vi "Control AlgorithmPID.vi"(5 "Motor to Control":dbl, 8 "Manual Control":bool, 9 "Angles In":dbl[](array[numeric]), 10 "JoystickIn":i16[](array[numeric])) -> (2 "Target Angles":dbl[](array[numeric]), 3 "MotorsOut":u16[](array[numeric]))   [LabVIEW 2012, in "ProcessorHelperFunctions.lvlib"]
uses:
  ProcessorHelperFunctions.lvlib
panel:
  in  "D gain":dbl
  in  "I Gain":dbl
  in  "Pgain":dbl=1.5
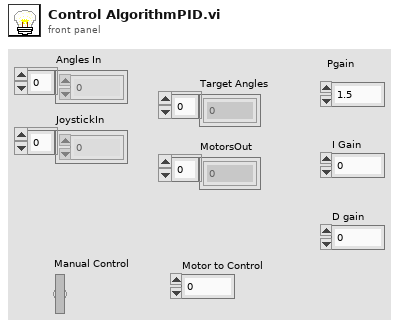
[diagram p1: front panel]
types:
  T1 = cluster{"JoystickIn[0]":i16, "JoystickIn[1]":i16, "JoystickIn[2]":i16, "JoystickIn[3]":i16, "JoystickIn[4]":i16, "JoystickIn[5]":i16, "JoystickIn[6]":i16, "JoystickIn[7]":i16, "JoystickIn[8]":i16, "JoystickIn[9]":i16}
  T2 = cluster{"Angles In[0]":dbl, "Angles In[1]":dbl, "Angles In[2]":dbl, "Angles In[3]":dbl}
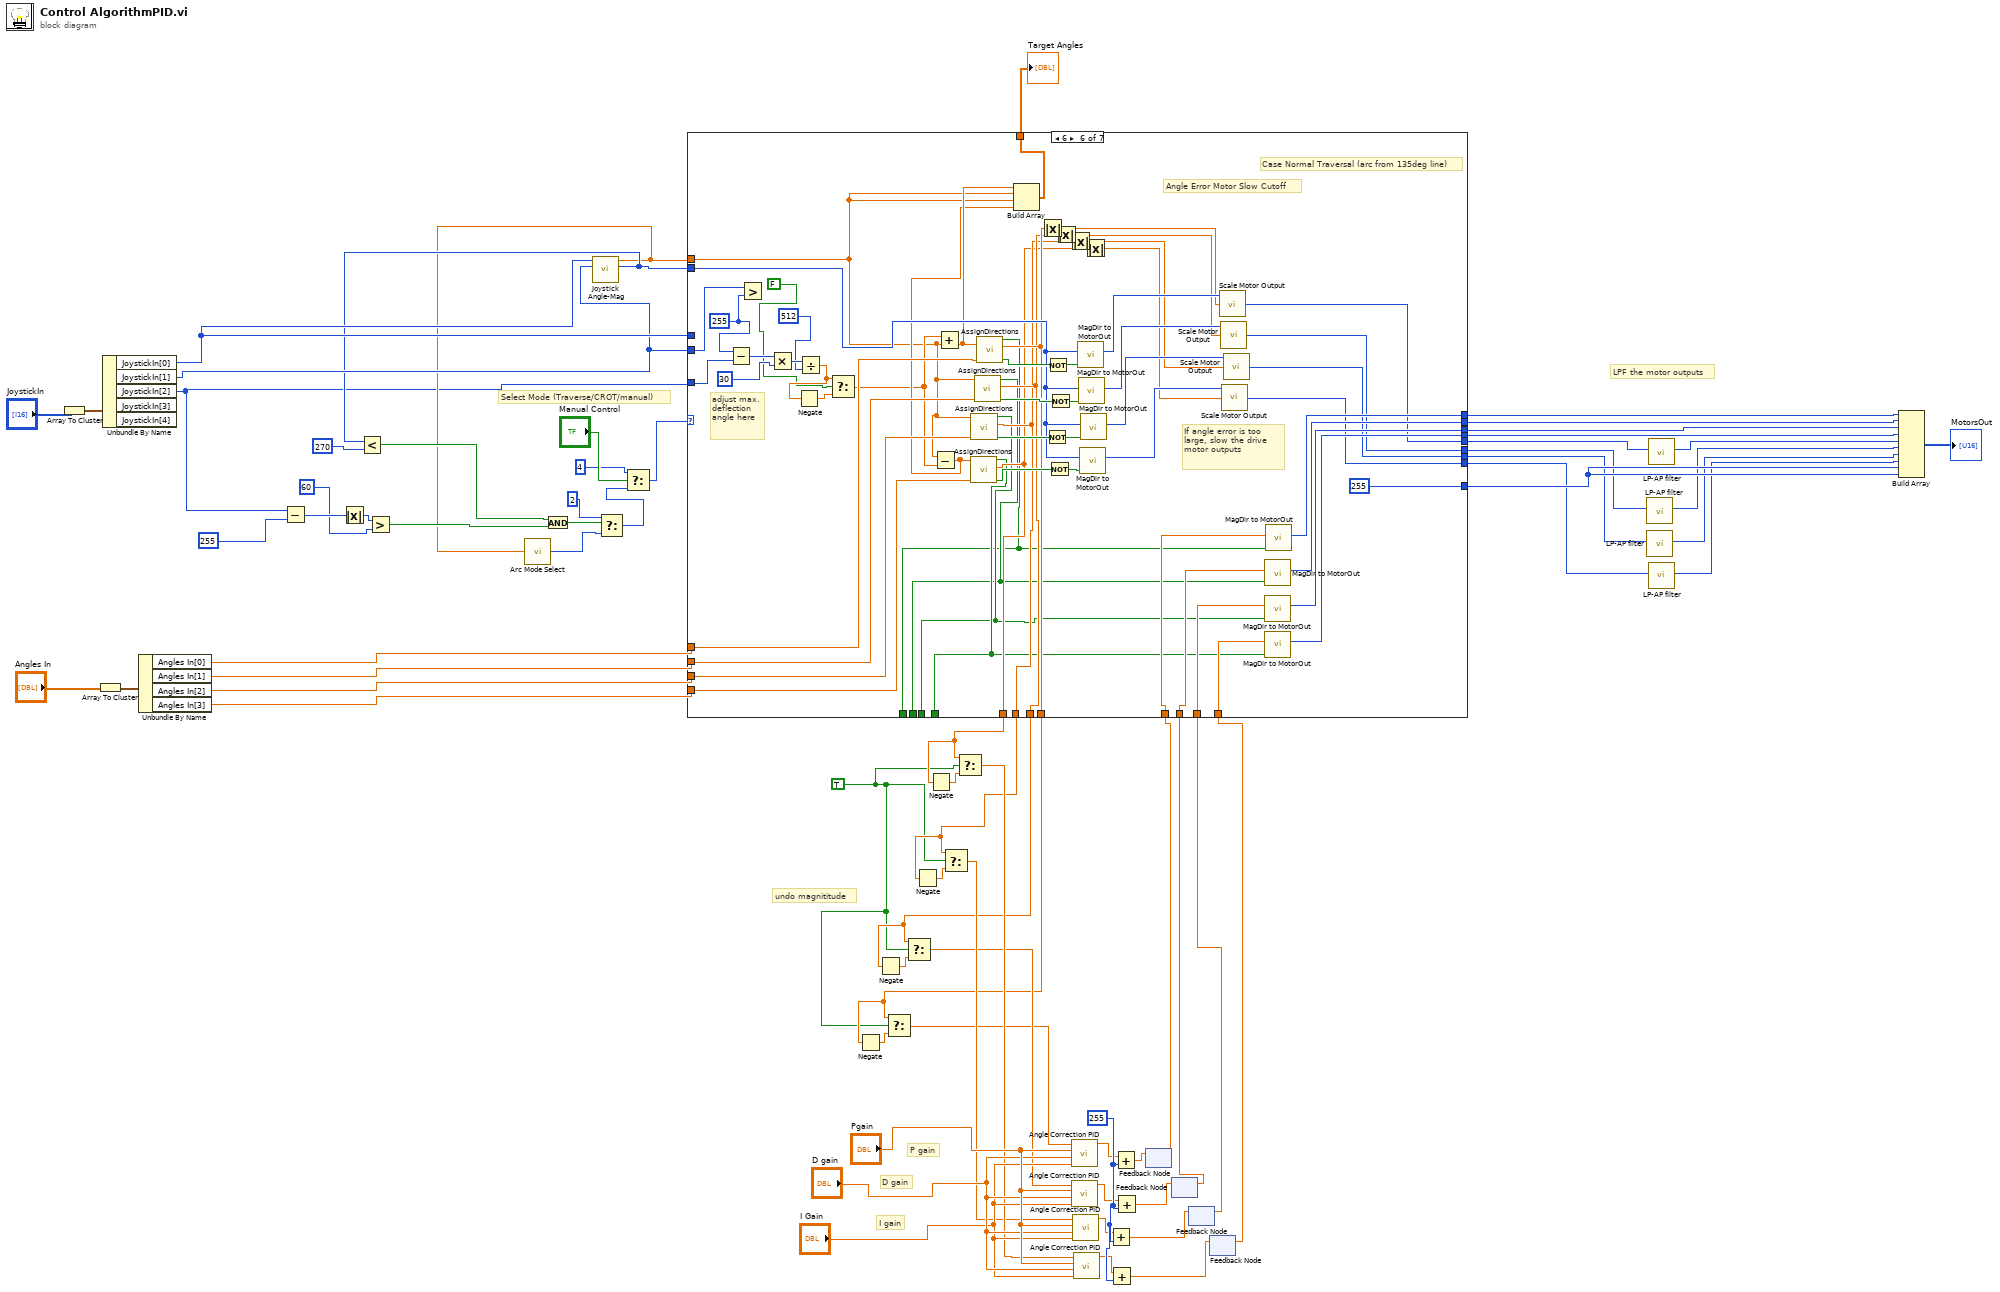
[diagram p0: block diagram]
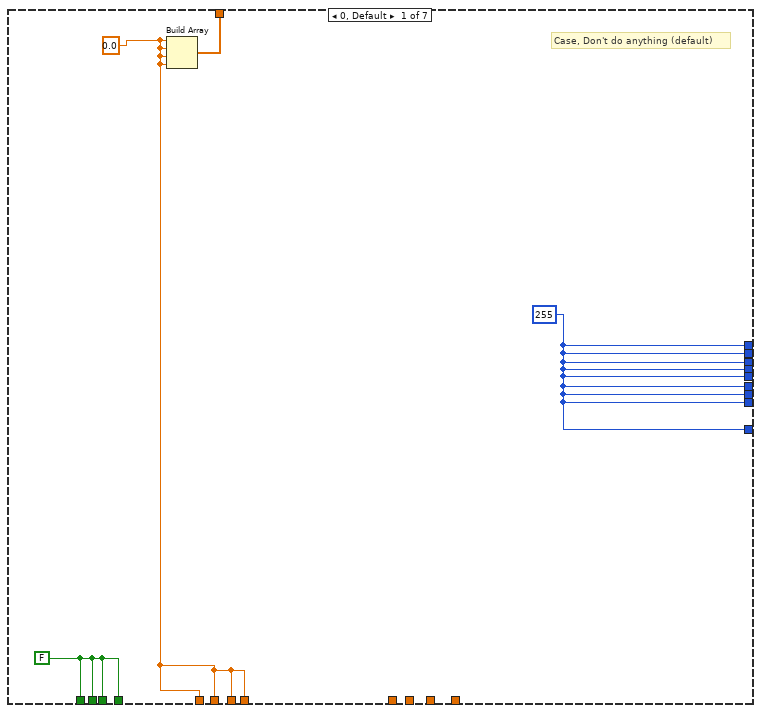
[diagram p2: hidden frame]
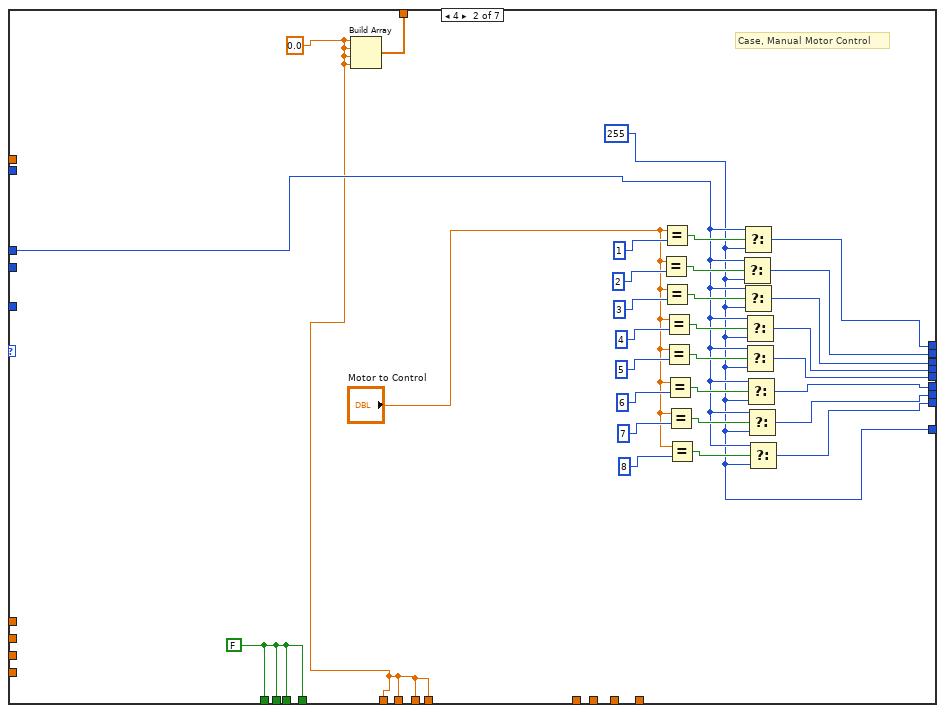
[diagram p3: hidden frame]
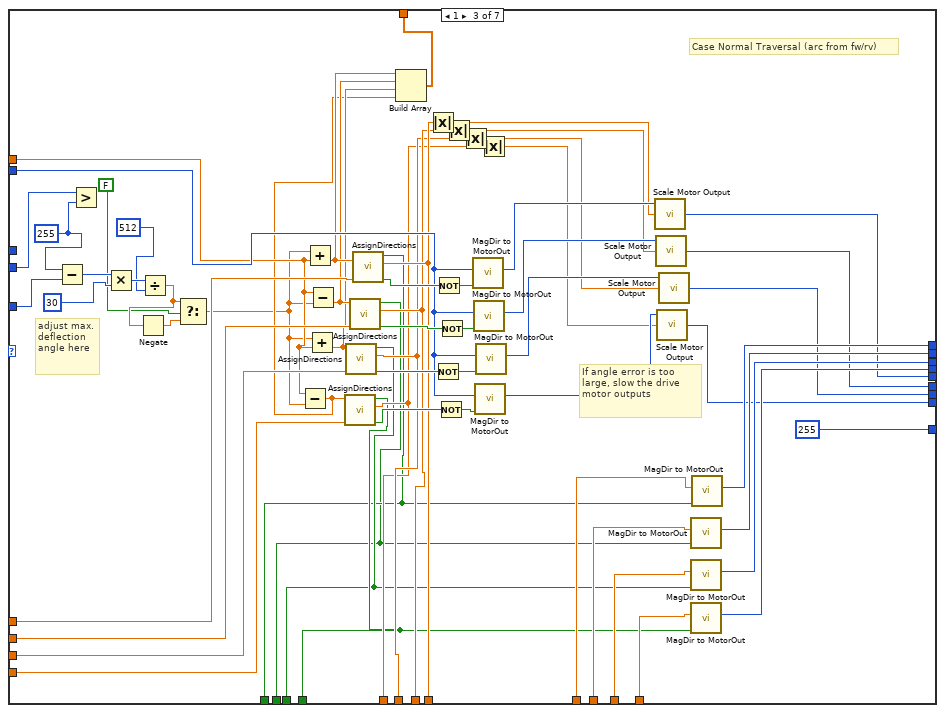
[diagram p4: hidden frame]
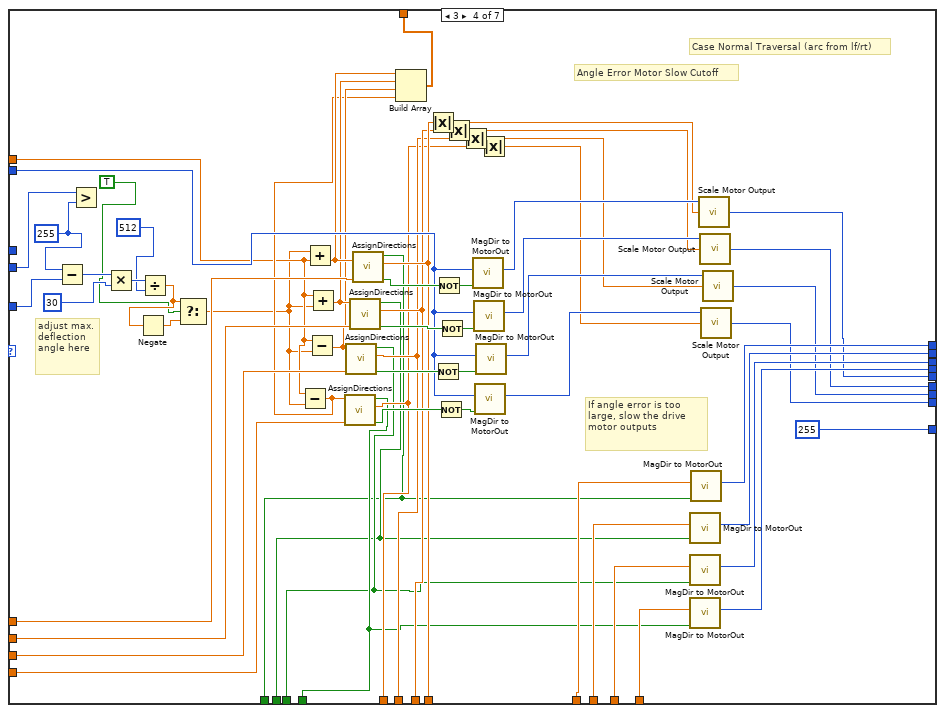
[diagram p5: hidden frame]
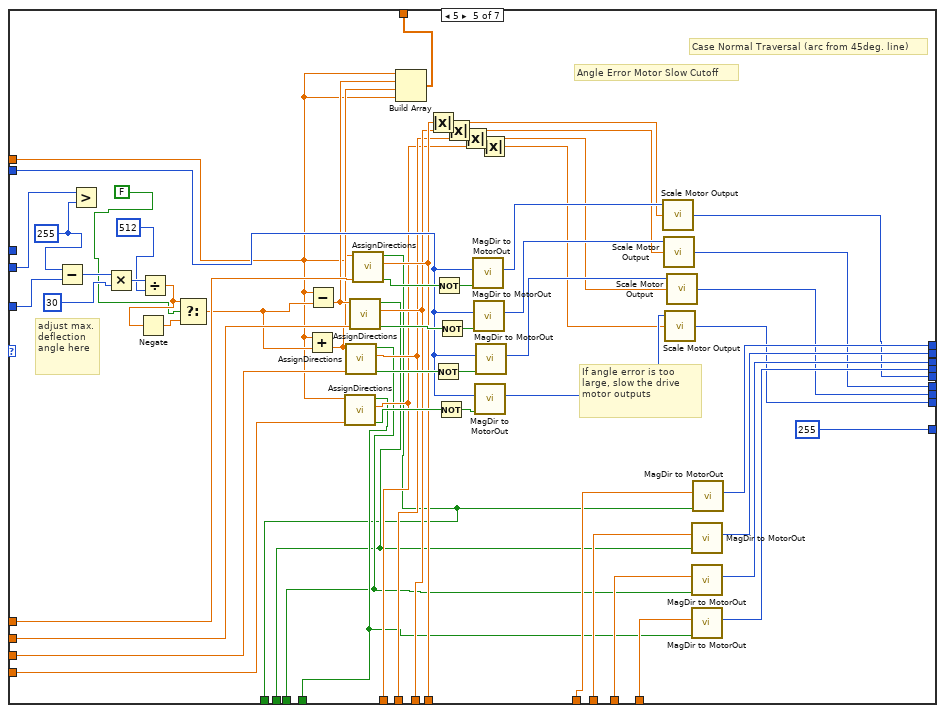
[diagram p6: hidden frame]
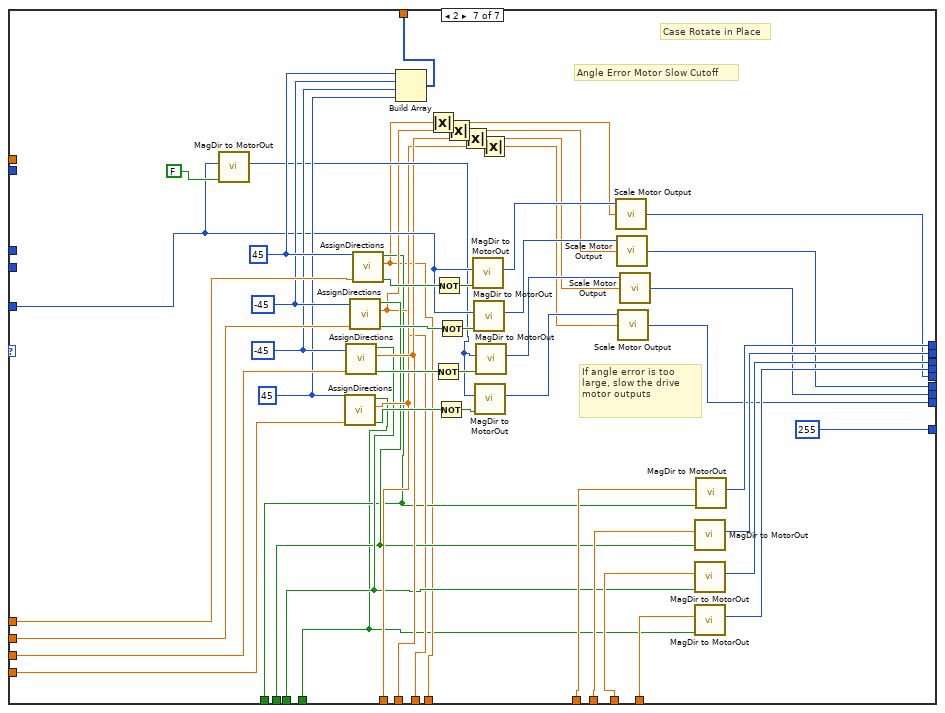
[diagram p7: hidden frame]
diagram:
  w6 = TRUE
  w30 = 255
  # "undo magnititude"
  # "I gain"
  # "D gain"
  # "P gain"
  # "LPF the motor outputs"
  # "Select Mode (Traverse/CROT/manual)"
  n1 = Array To Cluster(array="JoystickIn") -> (cluster=w70:T1)
  n2 = Array To Cluster(array="Angles In") -> (cluster=w63:T2)
  n3 = Unbundle By Name(w70) -> ("JoystickIn[0]"=w57:i16, "JoystickIn[1]"=w47:i16, "JoystickIn[2]"=w1:i16)  [unwired: 2 out]
  n4 = Unbundle By Name(w63) -> ("Angles In[0]"=w61:dbl, "Angles In[1]"=w60:dbl, "Angles In[2]"=w59:dbl, "Angles In[3]"=w58:dbl)
  n5 = Subtract(x=w1, y=255) -> (x-y=w54:i32)
  n6 = Absolute Value(x=w54) -> (abs(x)=w53:i32)
  n7 = Greater?(x=w53, y=60) -> (0:w49:bool)
  n8 = call "Joystick Angle-Mag.vi"("Yaxis"=w47, "Xaxis"=w57) -> ("Mag"=w33:i16, "Angle"=w31:dbl)  [unwired: 8 in]
  n9 = Less?(x=w33, y=270) -> (x < y?=w48:bool)
  n10 = call "Arc Mode Select.vi"("Angle"=w31) -> ("Mode"=w32:u8)
  n11 = And(x=w48, y=w49) -> (x .and. y?=w50:bool)
  n12 = Select(t=2, s=w50, f=w32) -> (s? t:f=w44:i32)
  n13 = Select(t=4, s="Manual Control", f=w44) -> (s? t:f=w45:i32)
  n14 = feedback #1() -> (w5:dbl)  [unwired: 1 in]
  n15 = feedback #2() -> (w4:dbl)  [unwired: 1 in]
  n16 = feedback #3() -> (w3:dbl)  [unwired: 1 in]
  n17 = feedback #4() -> (w2:dbl)  [unwired: 1 in]
  n18 = case shown="6" w45 {
    tunnel: [w75 w102 w160 w219 w276 w333 w382] -> w68
    tunnel: [w75 w86 w159 w218 w275 w332 w381] -> w67
    tunnel: [w75 w85 w158 w217 w274 w331 w380] -> w66
    tunnel: [w75 w84 w157 w216 w273 w330 w379] -> w65
    tunnel: [w75 w79 255 255 255 255 255] -> w64
    tunnel: [w75 w83 w110 w169 w227 w285 w343] -> w41
    tunnel: [w75 w82 w109 w168 w224 w284 w342] -> w39
    tunnel: [w75 w81 w108 w167 w226 w283 w345] -> w37
    tunnel: [w75 w80 w107 w166 w225 w282 w344] -> w35
    tunnel: w61 -> [_ _ w147 w206 w263 w320 w369]
    tunnel: w60 -> [_ _ w146 w205 w262 w319 w368]
    tunnel: w59 -> [_ _ w145 w204 w261 w318 w367]
    tunnel: w58 -> [_ _ w144 w203 w260 w317 w366]
    tunnel: w31 -> [_ _ w136 w187 w245 w303 _]
    tunnel: w33 -> [_ _ w143 w202 w259 w316 _]
    tunnel: w57 -> [_ w87 _ _ _ _ _]
    tunnel: w47 -> [_ _ w127 w188 w247 w302 _]
    tunnel: w1 -> [_ _ w141 w200 w257 w314 w360]
    tunnel: [w74 w105 w142 w201 w258 w315 w358] -> w56
    tunnel: [w73 w77 w125 w184 w243 w300 w339] -> w7
    tunnel: [w73 w77 w124 w183 w242 w299 w349] -> w11
    tunnel: [w73 w77 w123 w182 w241 w298 w357] -> w14
    tunnel: [w73 w77 w122 w181 w240 w297 w356] -> w17
    tunnel: w5 -> [_ _ w121 w180 w239 w296 w355]
    tunnel: w4 -> [_ _ w120 w179 w238 w295 w354]
    tunnel: w3 -> [_ _ w119 w178 w237 w294 w353]
    tunnel: w2 -> [_ _ w118 w177 w236 w293 w352]
    tunnel: [w72 w76 w117 w176 w235 w292 w338] -> _
    tunnel: [w72 w76 w116 w175 w234 w291 w351] -> _
    tunnel: [w72 w76 w114 w174 w233 w290 w350] -> _
    tunnel: [w72 w76 w115 w173 w232 w289 w348] -> _
    frame 0, Default {
      w72 = FALSE
      w73 = 0.0
      w75 = 255
      # "Case, Don't do anything (default)"
      n19 = Build Array(w73, w73, w73, w73) -> (w74:dbl[])
    }
    frame 4 {
      w76 = FALSE
      w79 = 255
      w77 = 0.0
      # "Case, Manual Motor Control"
      n20 = Build Array(w77, w77, w77, w77) -> (w105:dbl[])
      n21 = Equal?(x="Motor to Control", y=2) -> (x = y?=w100:bool)
      n22 = Equal?(x="Motor to Control", y=1) -> (x = y?=w103:bool)
      n23 = Equal?(x="Motor to Control", y=3) -> (x = y?=w98:bool)
      n24 = Equal?(x="Motor to Control", y=4) -> (x = y?=w96:bool)
      n25 = Equal?(x="Motor to Control", y=5) -> (x = y?=w94:bool)
      n26 = Equal?(x="Motor to Control", y=6) -> (x = y?=w92:bool)
      n27 = Equal?(x="Motor to Control", y=7) -> (x = y?=w90:bool)
      n28 = Equal?(x="Motor to Control", y=8) -> (x = y?=w88:bool)
      n29 = Select(t=w87, s=w100, f=w79) -> (s? t:f=w86:i32)
      n30 = Select(t=w87, s=w103, f=w79) -> (s? t:f=w102:i32)
      n31 = Select(t=w87, s=w98, f=w79) -> (s? t:f=w85:i32)
      n32 = Select(t=w87, s=w96, f=w79) -> (s? t:f=w84:i32)
      n33 = Select(t=w87, s=w94, f=w79) -> (s? t:f=w83:i32)
      n34 = Select(t=w87, s=w92, f=w79) -> (s? t:f=w82:i32)
      n35 = Select(t=w87, s=w90, f=w79) -> (s? t:f=w81:i32)
      n36 = Select(t=w87, s=w88, f=w79) -> (s? t:f=w80:i32)
    }
    frame 1 {
      w128 = 255
      # "adjust max. deflection angle here"
      # "Case Normal Traversal (arc from fw/rv)"
      # "If angle error is too large, slow the drive motor outputs"
      n37 = Subtract(x=w128, y=w141) -> (x-y=w139:i32)
      n38 = Greater?(x=w127, y=w128) -> ()  [unwired: 1 out]
      n39 = Multiply(x=w139, y=30) -> (x*y=w140:i32)
      n40 = Divide(x=w140, y=512) -> (x/y=w129:dbl)
      n41 = Negate(x=w129) -> (-x=w130:dbl)
      n42 = Select(t=w129, s=FALSE, f=w130) -> (s? t:f=w131:dbl)
      n43 = Subtract(x=w136, y=w131) -> (x-y=w132:dbl)
      n44 = Add(x=w131, y=w136) -> (x+y=w135:dbl)
      n45 = Add(x=w131, y=w136) -> (x+y=w133:dbl)
      n46 = Subtract(x=w136, y=w131) -> (x-y=w134:dbl)
      n47 = call "AssignDirections.vi"("Actual Angle"=w144, "Target Angle"=w132) -> ("Reverse Wheel Direction"=w161:bool, "Lowest Angle Error"=w122:dbl, "Turn Clockwise"=w117:bool)  [unwired: 7 in]
      n48 = call "AssignDirections.vi"("Actual Angle"=w145, "Target Angle"=w133) -> ("Reverse Wheel Direction"=w162:bool, "Lowest Angle Error"=w123:dbl, "Turn Clockwise"=w116:bool)  [unwired: 7 in]
      n49 = call "AssignDirections.vi"("Actual Angle"=w146, "Target Angle"=w134) -> ("Reverse Wheel Direction"=w163:bool, "Lowest Angle Error"=w124:dbl, "Turn Clockwise"=w114:bool)  [unwired: 7 in]
      n50 = call "AssignDirections.vi"("Actual Angle"=w147, "Target Angle"=w135) -> ("Reverse Wheel Direction"=w164:bool, "Lowest Angle Error"=w125:dbl, "Turn Clockwise"=w115:bool)  [unwired: 7 in]
      n51 = Build Array(w135, w134, w133, w132) -> (w142:dbl[])
      n52 = Absolute Value(x=w125) -> (abs(x)=w113:dbl)
      n53 = Not(x=w162) -> (.not. x?=w150:bool)
      n54 = Not(x=w164) -> (.not. x?=w148:bool)
      n55 = Not(x=w161) -> (.not. x?=w151:bool)
      n56 = Not(x=w163) -> (.not. x?=w149:bool)
      n57 = Absolute Value(x=w124) -> (abs(x)=w106:dbl)
      n58 = Absolute Value(x=w123) -> (abs(x)=w112:dbl)
      n59 = call "MagDir to MotorOut.vi"("Fwd. Dir?"=w148, "Input"=w143) -> ("Output"=w155:i16)  [unwired: 9 in]
      n60 = call "MagDir to MotorOut.vi"("Fwd. Dir?"=w149, "Input"=w143) -> ("Output"=w154:i16)  [unwired: 9 in]
      n61 = call "MagDir to MotorOut.vi"("Fwd. Dir?"=w151, "Input"=w143) -> ("Output"=w152:i16)  [unwired: 9 in]
      n62 = call "MagDir to MotorOut.vi"("Fwd. Dir?"=w150, "Input"=w143) -> ("Output"=w153:i16)  [unwired: 9 in]
      n63 = Absolute Value(x=w122) -> (abs(x)=w111:dbl)
      n64 = call "Scale Motor Output.vi"("Error Input"=w113, "Motor Input"=w155) -> ("Output"=w110:u32)  [unwired: 1 in]
      n65 = call "Scale Motor Output.vi"("Error Input"=w106, "Motor Input"=w154) -> ("Output"=w109:u32)  [unwired: 1 in]
      n66 = call "Scale Motor Output.vi"("Error Input"=w111, "Motor Input"=w152) -> ("Output"=w107:u32)  [unwired: 1 in]
      n67 = call "Scale Motor Output.vi"("Error Input"=w112, "Motor Input"=w153) -> ("Output"=w108:u32)  [unwired: 1 in]
      n68 = call "MagDir to MotorOut.vi"("Fwd. Dir?"=w114, "Input"=w120) -> ("Output"=w159:i16)  [unwired: 9 in]
      n69 = call "MagDir to MotorOut.vi"("Fwd. Dir?"=w116, "Input"=w119) -> ("Output"=w158:i16)  [unwired: 9 in]
      n70 = call "MagDir to MotorOut.vi"("Fwd. Dir?"=w117, "Input"=w118) -> ("Output"=w157:i16)  [unwired: 9 in]
      n71 = call "MagDir to MotorOut.vi"("Fwd. Dir?"=w115, "Input"=w121) -> ("Output"=w160:i16)  [unwired: 9 in]
    }
    frame 3 {
      w189 = 255
      # "adjust max. deflection angle here"
      # "Case Normal Traversal (arc from lf/rt)"
      # "Angle Error Motor Slow Cutoff"
      # "If angle error is too large, slow the drive motor outputs"
      n72 = Subtract(x=w189, y=w200) -> (x-y=w198:i32)
      n73 = Greater?(x=w188, y=w189) -> ()  [unwired: 1 out]
      n74 = Multiply(x=w198, y=30) -> (x*y=w199:i32)
      n75 = Divide(x=w199, y=512) -> (x/y=w190:dbl)
      n76 = Negate(x=w190) -> (-x=w191:dbl)
      n77 = Select(t=w190, s=TRUE, f=w191) -> (s? t:f=w186:dbl)
      n78 = Subtract(x=w187, y=w186) -> (x-y=w192:dbl)
      n79 = Add(x=w186, y=w187) -> (x+y=w195:dbl)
      n80 = Subtract(x=w187, y=w186) -> (x-y=w193:dbl)
      n81 = Add(x=w187, y=w186) -> (x+y=w194:dbl)
      n82 = call "AssignDirections.vi"("Actual Angle"=w203, "Target Angle"=w192) -> ("Reverse Wheel Direction"=w220:bool, "Lowest Angle Error"=w181:dbl, "Turn Clockwise"=w176:bool)  [unwired: 7 in]
      n83 = call "AssignDirections.vi"("Actual Angle"=w204, "Target Angle"=w193) -> ("Reverse Wheel Direction"=w221:bool, "Lowest Angle Error"=w182:dbl, "Turn Clockwise"=w175:bool)  [unwired: 7 in]
      n84 = call "AssignDirections.vi"("Actual Angle"=w205, "Target Angle"=w194) -> ("Reverse Wheel Direction"=w222:bool, "Lowest Angle Error"=w183:dbl, "Turn Clockwise"=w174:bool)  [unwired: 7 in]
      n85 = call "AssignDirections.vi"("Actual Angle"=w206, "Target Angle"=w195) -> ("Reverse Wheel Direction"=w223:bool, "Lowest Angle Error"=w184:dbl, "Turn Clockwise"=w173:bool)  [unwired: 7 in]
      n86 = Build Array(w195, w194, w193, w192) -> (w201:dbl[])
      n87 = Absolute Value(x=w184) -> (abs(x)=w172:dbl)
      n88 = Not(x=w221) -> (.not. x?=w209:bool)
      n89 = Not(x=w223) -> (.not. x?=w207:bool)
      n90 = Not(x=w220) -> (.not. x?=w210:bool)
      n91 = Not(x=w222) -> (.not. x?=w208:bool)
      n92 = Absolute Value(x=w183) -> (abs(x)=w171:dbl)
      n93 = Absolute Value(x=w182) -> (abs(x)=w170:dbl)
      n94 = call "MagDir to MotorOut.vi"("Fwd. Dir?"=w207, "Input"=w202) -> ("Output"=w214:i16)  [unwired: 9 in]
      n95 = call "MagDir to MotorOut.vi"("Fwd. Dir?"=w208, "Input"=w202) -> ("Output"=w213:i16)  [unwired: 9 in]
      n96 = call "MagDir to MotorOut.vi"("Fwd. Dir?"=w210, "Input"=w202) -> ("Output"=w211:i16)  [unwired: 9 in]
      n97 = call "MagDir to MotorOut.vi"("Fwd. Dir?"=w209, "Input"=w202) -> ("Output"=w212:i16)  [unwired: 9 in]
      n98 = Absolute Value(x=w181) -> (abs(x)=w165:dbl)
      n99 = call "MagDir to MotorOut.vi"("Fwd. Dir?"=w174, "Input"=w179) -> ("Output"=w218:i16)  [unwired: 9 in]
      n100 = call "MagDir to MotorOut.vi"("Fwd. Dir?"=w175, "Input"=w178) -> ("Output"=w217:i16)  [unwired: 9 in]
      n101 = call "MagDir to MotorOut.vi"("Fwd. Dir?"=w176, "Input"=w177) -> ("Output"=w216:i16)  [unwired: 9 in]
      n102 = call "MagDir to MotorOut.vi"("Fwd. Dir?"=w173, "Input"=w180) -> ("Output"=w219:i16)  [unwired: 9 in]
      n103 = call "Scale Motor Output.vi"("Error Input"=w172, "Motor Input"=w214) -> ("Output"=w169:u32)  [unwired: 1 in]
      n104 = call "Scale Motor Output.vi"("Error Input"=w171, "Motor Input"=w213) -> ("Output"=w168:u32)  [unwired: 1 in]
      n105 = call "Scale Motor Output.vi"("Error Input"=w165, "Motor Input"=w211) -> ("Output"=w166:u32)  [unwired: 1 in]
      n106 = call "Scale Motor Output.vi"("Error Input"=w170, "Motor Input"=w212) -> ("Output"=w167:u32)  [unwired: 1 in]
    }
    frame 5 {
      w248 = 255
      # "adjust max. deflection angle here"
      # "Case Normal Traversal (arc from 45deg. line)"
      # "Angle Error Motor Slow Cutoff"
      # "If angle error is too large, slow the drive motor outputs"
      n107 = Subtract(x=w248, y=w257) -> (x-y=w255:i32)
      n108 = Greater?(x=w247, y=w248) -> ()  [unwired: 1 out]
      n109 = Multiply(x=w255, y=30) -> (x*y=w256:i32)
      n110 = Divide(x=w256, y=512) -> (x/y=w249:dbl)
      n111 = Negate(x=w249) -> (-x=w250:dbl)
      n112 = Select(t=w249, s=FALSE, f=w250) -> (s? t:f=w246:dbl)
      n113 = Add(x=w245, y=w246) -> (x+y=w251:dbl)
      n114 = Subtract(x=w245, y=w246) -> (x-y=w252:dbl)
      n115 = call "AssignDirections.vi"("Actual Angle"=w260, "Target Angle"=w245) -> ("Reverse Wheel Direction"=w277:bool, "Lowest Angle Error"=w240:dbl, "Turn Clockwise"=w235:bool)  [unwired: 7 in]
      n116 = call "AssignDirections.vi"("Actual Angle"=w261, "Target Angle"=w251) -> ("Reverse Wheel Direction"=w278:bool, "Lowest Angle Error"=w241:dbl, "Turn Clockwise"=w234:bool)  [unwired: 7 in]
      n117 = call "AssignDirections.vi"("Actual Angle"=w262, "Target Angle"=w252) -> ("Reverse Wheel Direction"=w279:bool, "Lowest Angle Error"=w242:dbl, "Turn Clockwise"=w233:bool)  [unwired: 7 in]
      n118 = call "AssignDirections.vi"("Actual Angle"=w263, "Target Angle"=w245) -> ("Reverse Wheel Direction"=w280:bool, "Lowest Angle Error"=w243:dbl, "Turn Clockwise"=w232:bool)  [unwired: 7 in]
      n119 = Build Array(w245, w252, w251, w245) -> (w258:dbl[])
      n120 = Absolute Value(x=w243) -> (abs(x)=w231:dbl)
      n121 = Not(x=w278) -> (.not. x?=w266:bool)
      n122 = Not(x=w280) -> (.not. x?=w264:bool)
      n123 = Not(x=w277) -> (.not. x?=w267:bool)
      n124 = Not(x=w279) -> (.not. x?=w265:bool)
      n125 = Absolute Value(x=w242) -> (abs(x)=w230:dbl)
      n126 = Absolute Value(x=w241) -> (abs(x)=w229:dbl)
      n127 = call "MagDir to MotorOut.vi"("Fwd. Dir?"=w264, "Input"=w259) -> ("Output"=w271:i16)  [unwired: 9 in]
      n128 = call "MagDir to MotorOut.vi"("Fwd. Dir?"=w265, "Input"=w259) -> ("Output"=w270:i16)  [unwired: 9 in]
      n129 = call "MagDir to MotorOut.vi"("Fwd. Dir?"=w267, "Input"=w259) -> ("Output"=w268:i16)  [unwired: 9 in]
      n130 = call "MagDir to MotorOut.vi"("Fwd. Dir?"=w266, "Input"=w259) -> ("Output"=w269:i16)  [unwired: 9 in]
      n131 = Absolute Value(x=w240) -> (abs(x)=w228:dbl)
      n132 = call "Scale Motor Output.vi"("Error Input"=w231, "Motor Input"=w271) -> ("Output"=w227:u32)  [unwired: 1 in]
      n133 = call "Scale Motor Output.vi"("Error Input"=w230, "Motor Input"=w270) -> ("Output"=w224:u32)  [unwired: 1 in]
      n134 = call "Scale Motor Output.vi"("Error Input"=w228, "Motor Input"=w268) -> ("Output"=w225:u32)  [unwired: 1 in]
      n135 = call "Scale Motor Output.vi"("Error Input"=w229, "Motor Input"=w269) -> ("Output"=w226:u32)  [unwired: 1 in]
      n136 = call "MagDir to MotorOut.vi"("Fwd. Dir?"=w233, "Input"=w238) -> ("Output"=w275:i16)  [unwired: 9 in]
      n137 = call "MagDir to MotorOut.vi"("Fwd. Dir?"=w234, "Input"=w237) -> ("Output"=w274:i16)  [unwired: 9 in]
      n138 = call "MagDir to MotorOut.vi"("Fwd. Dir?"=w235, "Input"=w236) -> ("Output"=w273:i16)  [unwired: 9 in]
      n139 = call "MagDir to MotorOut.vi"("Fwd. Dir?"=w232, "Input"=w239) -> ("Output"=w276:i16)  [unwired: 9 in]
    }
    frame 6 {
      w304 = 255
      # "adjust max. deflection angle here"
      # "Case Normal Traversal (arc from 135deg line)"
      # "Angle Error Motor Slow Cutoff"
      # "If angle error is too large, slow the drive motor outputs"
      n140 = Subtract(x=w304, y=w314) -> (x-y=w312:i32)
      n141 = Greater?(x=w302, y=w304) -> ()  [unwired: 1 out]
      n142 = Multiply(x=w312, y=30) -> (x*y=w313:i32)
      n143 = Divide(x=w313, y=512) -> (x/y=w305:dbl)
      n144 = Negate(x=w305) -> (-x=w306:dbl)
      n145 = Select(t=w305, s=FALSE, f=w306) -> (s? t:f=w307:dbl)
      n146 = Subtract(x=w303, y=w307) -> (x-y=w308:dbl)
      n147 = Add(x=w307, y=w303) -> (x+y=w309:dbl)
      n148 = call "AssignDirections.vi"("Actual Angle"=w317, "Target Angle"=w308) -> ("Reverse Wheel Direction"=w334:bool, "Lowest Angle Error"=w297:dbl, "Turn Clockwise"=w292:bool)  [unwired: 7 in]
      n149 = call "AssignDirections.vi"("Actual Angle"=w318, "Target Angle"=w303) -> ("Reverse Wheel Direction"=w335:bool, "Lowest Angle Error"=w298:dbl, "Turn Clockwise"=w291:bool)  [unwired: 7 in]
      n150 = call "AssignDirections.vi"("Actual Angle"=w319, "Target Angle"=w303) -> ("Reverse Wheel Direction"=w336:bool, "Lowest Angle Error"=w299:dbl, "Turn Clockwise"=w290:bool)  [unwired: 7 in]
      n151 = call "AssignDirections.vi"("Actual Angle"=w320, "Target Angle"=w309) -> ("Reverse Wheel Direction"=w337:bool, "Lowest Angle Error"=w300:dbl, "Turn Clockwise"=w289:bool)  [unwired: 7 in]
      n152 = Build Array(w309, w303, w303, w308) -> (w315:dbl[])
      n153 = Absolute Value(x=w300) -> (abs(x)=w288:dbl)
      n154 = Not(x=w335) -> (.not. x?=w323:bool)
      n155 = Not(x=w337) -> (.not. x?=w321:bool)
      n156 = Not(x=w334) -> (.not. x?=w324:bool)
      n157 = Not(x=w336) -> (.not. x?=w322:bool)
      n158 = Absolute Value(x=w299) -> (abs(x)=w281:dbl)
      n159 = Absolute Value(x=w298) -> (abs(x)=w287:dbl)
      n160 = call "MagDir to MotorOut.vi"("Fwd. Dir?"=w321, "Input"=w316) -> ("Output"=w328:i16)  [unwired: 9 in]
      n161 = call "MagDir to MotorOut.vi"("Fwd. Dir?"=w322, "Input"=w316) -> ("Output"=w327:i16)  [unwired: 9 in]
      n162 = call "MagDir to MotorOut.vi"("Fwd. Dir?"=w324, "Input"=w316) -> ("Output"=w325:i16)  [unwired: 9 in]
      n163 = call "MagDir to MotorOut.vi"("Fwd. Dir?"=w323, "Input"=w316) -> ("Output"=w326:i16)  [unwired: 9 in]
      n164 = Absolute Value(x=w297) -> (abs(x)=w286:dbl)
      n165 = call "Scale Motor Output.vi"("Error Input"=w288, "Motor Input"=w328) -> ("Output"=w285:u32)  [unwired: 1 in]
      n166 = call "Scale Motor Output.vi"("Error Input"=w281, "Motor Input"=w327) -> ("Output"=w284:u32)  [unwired: 1 in]
      n167 = call "Scale Motor Output.vi"("Error Input"=w286, "Motor Input"=w325) -> ("Output"=w282:u32)  [unwired: 1 in]
      n168 = call "Scale Motor Output.vi"("Error Input"=w287, "Motor Input"=w326) -> ("Output"=w283:u32)  [unwired: 1 in]
      n169 = call "MagDir to MotorOut.vi"("Fwd. Dir?"=w290, "Input"=w295) -> ("Output"=w332:i16)  [unwired: 9 in]
      n170 = call "MagDir to MotorOut.vi"("Fwd. Dir?"=w291, "Input"=w294) -> ("Output"=w331:i16)  [unwired: 9 in]
      n171 = call "MagDir to MotorOut.vi"("Fwd. Dir?"=w292, "Input"=w293) -> ("Output"=w330:i16)  [unwired: 9 in]
      n172 = call "MagDir to MotorOut.vi"("Fwd. Dir?"=w289, "Input"=w296) -> ("Output"=w333:i16)  [unwired: 9 in]
    }
    frame 2 {
      w362 = 45
      w363 = -45
      w364 = -45
      w365 = 45
      # "Case Rotate in Place"
      # "Angle Error Motor Slow Cutoff"
      # "If angle error is too large, slow the drive motor outputs"
      n173 = call "MagDir to MotorOut.vi"("Fwd. Dir?"=FALSE, "Input"=w360) -> ("Output"=w359:i16)  [unwired: 9 in]
      n174 = call "AssignDirections.vi"("Actual Angle"=w366, "Target Angle"=w362) -> ("Reverse Wheel Direction"=w383:bool, "Lowest Angle Error"=w356:dbl, "Turn Clockwise"=w338:bool)  [unwired: 7 in]
      n175 = call "AssignDirections.vi"("Actual Angle"=w367, "Target Angle"=w363) -> ("Reverse Wheel Direction"=w384:bool, "Lowest Angle Error"=w357:dbl, "Turn Clockwise"=w351:bool)  [unwired: 7 in]
      n176 = call "AssignDirections.vi"("Actual Angle"=w368, "Target Angle"=w364) -> ("Reverse Wheel Direction"=w385:bool, "Lowest Angle Error"=w349:dbl, "Turn Clockwise"=w350:bool)  [unwired: 7 in]
      n177 = call "AssignDirections.vi"("Actual Angle"=w369, "Target Angle"=w365) -> ("Reverse Wheel Direction"=w386:bool, "Lowest Angle Error"=w339:dbl, "Turn Clockwise"=w348:bool)  [unwired: 7 in]
      n178 = Build Array(w365, w364, w363, w362) -> (w358:i32[])
      n179 = Absolute Value(x=w339) -> (abs(x)=w347:dbl)
      n180 = Not(x=w384) -> (.not. x?=w372:bool)
      n181 = Not(x=w386) -> (.not. x?=w370:bool)
      n182 = Not(x=w383) -> (.not. x?=w373:bool)
      n183 = Not(x=w385) -> (.not. x?=w371:bool)
      n184 = Absolute Value(x=w349) -> (abs(x)=w346:dbl)
      n185 = Absolute Value(x=w357) -> (abs(x)=w341:dbl)
      n186 = call "MagDir to MotorOut.vi"("Fwd. Dir?"=w370, "Input"=w360) -> ("Output"=w377:i16)  [unwired: 9 in]
      n187 = call "MagDir to MotorOut.vi"("Fwd. Dir?"=w371, "Input"=w360) -> ("Output"=w376:i16)  [unwired: 9 in]
      n188 = call "MagDir to MotorOut.vi"("Fwd. Dir?"=w373, "Input"=w359) -> ("Output"=w374:i16)  [unwired: 9 in]
      n189 = call "MagDir to MotorOut.vi"("Fwd. Dir?"=w372, "Input"=w359) -> ("Output"=w375:i16)  [unwired: 9 in]
      n190 = Absolute Value(x=w356) -> (abs(x)=w340:dbl)
      n191 = call "Scale Motor Output.vi"("Error Input"=w347, "Motor Input"=w377) -> ("Output"=w343:u32)  [unwired: 1 in]
      n192 = call "Scale Motor Output.vi"("Error Input"=w346, "Motor Input"=w376) -> ("Output"=w342:u32)  [unwired: 1 in]
      n193 = call "Scale Motor Output.vi"("Error Input"=w340, "Motor Input"=w374) -> ("Output"=w344:u32)  [unwired: 1 in]
      n194 = call "Scale Motor Output.vi"("Error Input"=w341, "Motor Input"=w375) -> ("Output"=w345:u32)  [unwired: 1 in]
      n195 = call "MagDir to MotorOut.vi"("Fwd. Dir?"=w350, "Input"=w354) -> ("Output"=w381:i16)  [unwired: 9 in]
      n196 = call "MagDir to MotorOut.vi"("Fwd. Dir?"=w351, "Input"=w353) -> ("Output"=w380:i16)  [unwired: 9 in]
      n197 = call "MagDir to MotorOut.vi"("Fwd. Dir?"=w338, "Input"=w352) -> ("Output"=w379:i16)  [unwired: 9 in]
      n198 = call "MagDir to MotorOut.vi"("Fwd. Dir?"=w348, "Input"=w355) -> ("Output"=w382:i16)  [unwired: 9 in]
    }
  }
  "Target Angles" <- w56
  n199 = Negate(x=w7) -> (-x=w9:dbl)
  n200 = Negate(x=w11) -> (-x=w12:dbl)
  n201 = Select(t=w7, s=w6, f=w9) -> (s? t:f=w8:dbl)
  n202 = Select(t=w11, s=w6, f=w12) -> (s? t:f=w10:dbl)
  n203 = Negate(x=w14) -> (-x=w15:dbl)
  n204 = Negate(x=w17) -> (-x=w18:dbl)
  n205 = Select(t=w14, s=w6, f=w15) -> (s? t:f=w13:dbl)
  n206 = Select(t=w17, s=w6, f=w18) -> (s? t:f=w16:dbl)
  n207 = call "Angle Correction PID.vi"("I gain"="I Gain", "D gain"="D gain", "P gain"="Pgain", "Error In"=w8) -> ("Output"=w25:dbl)  [unwired: 7 in]
  n208 = call "Angle Correction PID.vi"("I gain"="I Gain", "D gain"="D gain", "P gain"="Pgain", "Error In"=w10) -> ("Output"=w24:dbl)  [unwired: 7 in]
  n209 = call "Angle Correction PID.vi"("I gain"="I Gain", "D gain"="D gain", "P gain"="Pgain", "Error In"=w13) -> ("Output"=w23:dbl)  [unwired: 7 in]
  n210 = call "Angle Correction PID.vi"("I gain"="I Gain", "D gain"="D gain", "P gain"="Pgain", "Error In"=w16) -> ("Output"=w22:dbl)  [unwired: 7 in]
  n211 = Add(x=w23, y=w30) -> (x+y=w27:dbl)
  n212 = Add(x=w22, y=w30) -> (x+y=w26:dbl)
  n213 = Add(x=w25, y=w30) -> (x+y=w29:dbl)
  n214 = Add(x=w24, y=w30) -> (x+y=w28:dbl)
  n215 = feedback-in #1(w29) -> ()
  n216 = feedback-in #2(w28) -> ()
  n217 = feedback-in #3(w27) -> ()
  n218 = feedback-in #4(w26) -> ()
  n219 = call "LP-AP filter.vi"("Input"=w39) -> ("Output"=w38:u16)  [unwired: 9 in, 1 out]
  n220 = call "LP-AP filter.vi"("Input"=w37) -> ("Output"=w36:u16)  [unwired: 9 in, 1 out]
  n221 = call "LP-AP filter.vi"("Input"=w41) -> ("Output"=w40:u16)  [unwired: 9 in, 1 out]
  n222 = call "LP-AP filter.vi"("Input"=w35) -> ("Output"=w34:u16)  [unwired: 9 in, 1 out]
  n223 = Build Array(w68, w67, w66, w65, w40, w38, w36, w34, w64, w64) -> (→"MotorsOut":i32[])
